vi "Finish.vi"   [LabVIEW 2015]
doc: "This VI is called just before exiting. It is expected to close I/O refnum, save collected data, etc."
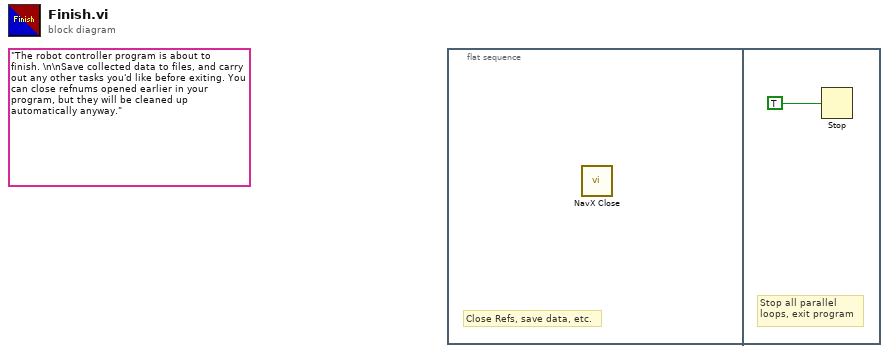
[diagram p0: block diagram]
diagram:
  (unwired) "The robot controller program is about to finish. \n\nSave collected data to files, and carry out any other tasks you'd like before exiting. You can close refnums opened earlier in your program, but they will be cleaned up automatically anyway."
  n1 = flat-sequence {
    frame #0 {
      # "Close Refs, save data, etc."
      n2 = call "NavX Close.vi"() -> ()  [unwired: 11 in, 1 out]
    }
    frame #1 {
      # "Stop all parallel\nloops, exit program"
      n3 = Stop(stop? (T)=TRUE ("Quit")) -> ()
    }
  }
